vi "SRX Read Velocity Sensor Data.vi"(7 "Target":dbl, 8 "Error":errorcluster, 11 "SRX Ref":T4) -> (0 "Error Out":errorcluster, 2 "Sensor Status Out":T1, 3 "SRX Ref Out":T4)   [LabVIEW 2020, in "Shooter_ACT.lvlib"]
uses:
  Shooter_ACT.lvlib
  <vilib>/Rock Robotics/WPI/MotorControl/WPI_MotorControlDeviceRef.ctl
  <vilib>/Rock Robotics/WPI/MotorControl/WPI_MotorControlType.ctl
  <vilib>/Rock Robotics/SystemInterfaces/DIO/FPGA_DIOPWMChannel.ctl
  <vilib>/Rock Robotics/WPI/PWM/WPI_PWMDeadband.ctl
  <vilib>/Rock Robotics/SystemInterfaces/DIO/FPGA_DIOChannel.ctl
  Cluster_Speed Sensor Values.ctl
  Cluster_Velocity Values.ctl
  Cluster_Voltage Values.ctl
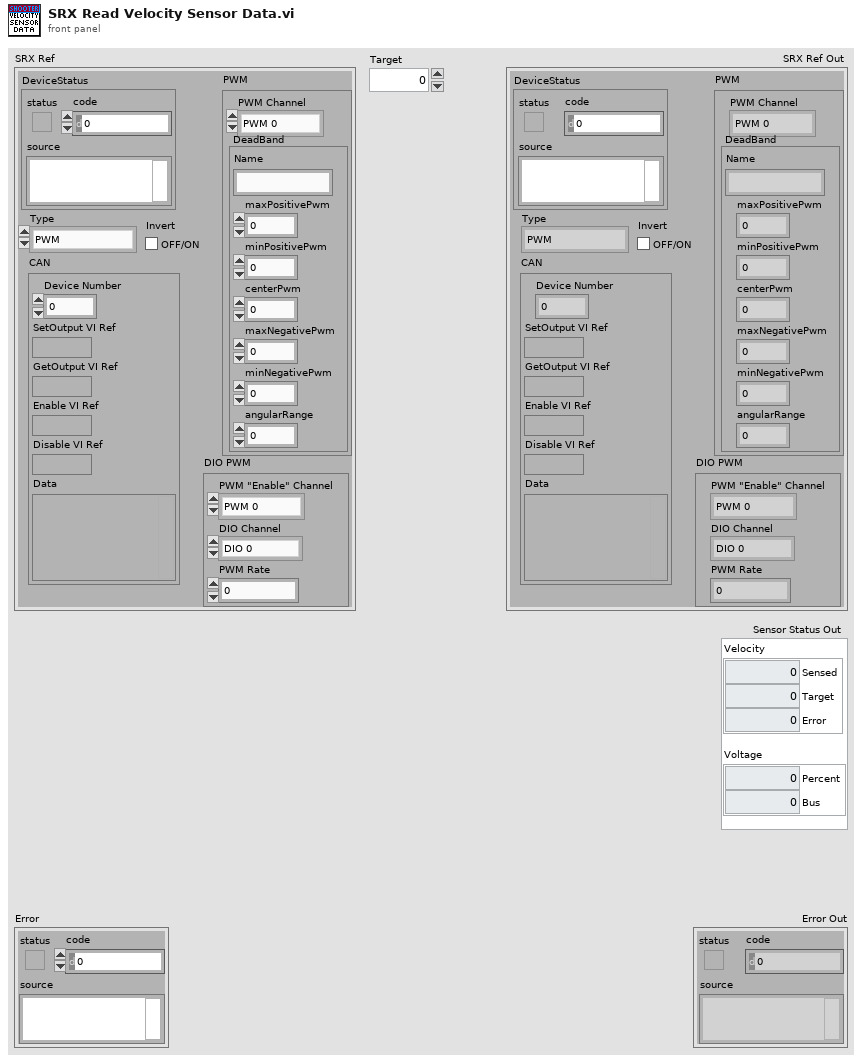
[diagram p1: front panel]
types:
  T1 = typedef "Cluster_Speed Sensor Values.ctl" = cluster{"Velocity":T2, "Voltage":T3}
  T2 = typedef "Shooter_ACT.lvlib/Cluster_Velocity Values.ctl" = cluster{"Sensed":dbl, "Target":dbl, "Error":dbl}
  T3 = typedef "Shooter_ACT.lvlib/Cluster_Voltage Values.ctl" = cluster{"Percent":dbl, "Bus":dbl}
  T4 = typedef "WPI_MotorControlDeviceRef.ctl" = cluster{"DeviceStatus":errorcluster, "Type":T5, "PWM":cluster{"PWM Channel":T6, "DeadBand":T7}, "CAN":cluster{"Device Number":u8, "SetOutput VI Ref":variant, "GetOutput VI Ref":variant, "Enable VI Ref":variant, "Disable VI Ref":variant, "Data":variant}, "Invert":bool, "DIO PWM":cluster{"PWM \"Enable\" Channel":T6, "DIOChannel":T8, "PWM Rate":dbl}}
  T5 = typedef "WPI_MotorControlType.ctl" = enum16{"PWM", "CAN", "DIO PWM"}
  T6 = typedef "FPGA_DIOPWMChannel.ctl" = enum8{"PWM 0", "PWM 1", "PWM 2", "PWM 3", "PWM 4", "PWM 5", "PWM 6", "PWM 7", "PWM 8", "PWM 9", "PWM MXP 0", "PWM MXP 1", "PWM MXP 2", "PWM MXP 3", "PWM MXP 4", "PWM MXP 5", "PWM MXP 6", "PWM MXP 7", "PWM MXP 8", "PWM MXP 9", "Invalid"}
  T7 = typedef "WPI_PWMDeadband.ctl" = cluster{"Name":string, "maxPositivePwm":i32, "minPositivePwm":i32, "centerPwm":i32, "maxNegativePwm":i32, "minNegativePwm":i32, "angularRange":u16}
  T8 = typedef "FPGA_DIOChannel.ctl" = enum8{"DIO 0", "DIO 1", "DIO 2", "DIO 3", "DIO 4", "DIO 5", "DIO 6", "DIO 7", "DIO 8", "DIO 9", "DIO MXP 0", "DIO MXP 1", "DIO MXP 2", "DIO MXP 3", "DIO MXP 4", "DIO MXP 5", "DIO MXP 6", "DIO MXP 7", "DIO MXP 8", "DIO MXP 9", "DIO MXP 10", "DIO MXP 11", "DIO MXP 12", "DIO MXP 13", "DIO MXP 14", "DIO MXP 15", "SPI Port CS1", "SPI Port CS2", "SPI Port CS3", "SPI Port MISO", "SPI Port MOSI", "Invalid"}
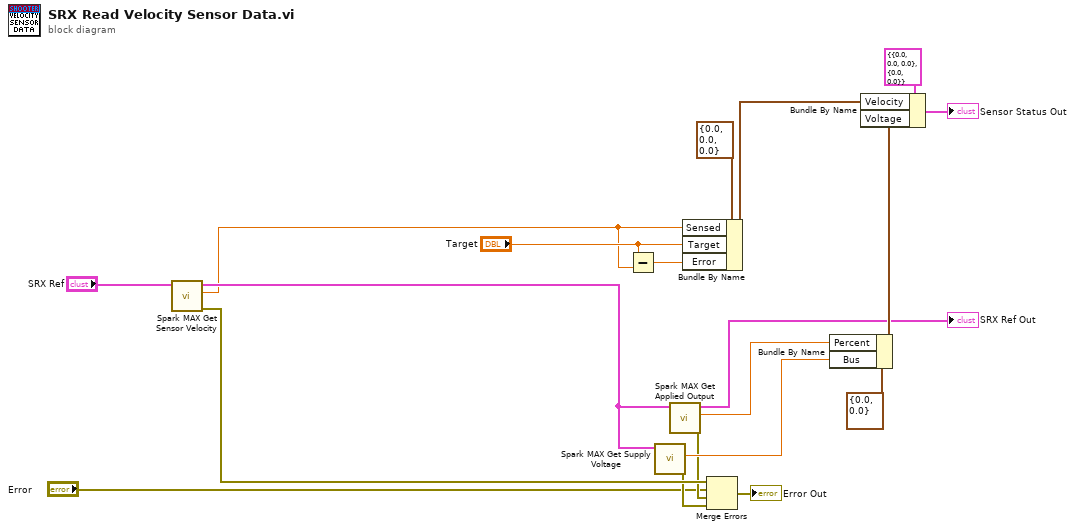
[diagram p0: block diagram]
diagram:
  n1 = call <vilib>:"Spark MAX Get Sensor Velocity.vi"("MotorControlDevRef in"="SRX Ref") -> ("error out"=w11:errorcluster, "Sensor Velocity"=w2:dbl, "MotorControlDevRef out"=w5:T4)  [unwired: 7 in, 1 out]
  n2 = Subtract(x="Target", y=w2) -> (x-y=w1:dbl)
  n3 = call <vilib>:"Spark MAX Get Supply Voltage.vi"("MotorControlDevRef in"=w5) -> ("error out"=w7:errorcluster, "Voltage"=w9:dbl)  [unwired: 7 in, 2 out]
  n4 = call <vilib>:"Spark MAX Get Applied Output.vi"("MotorControlDevRef in"=w5) -> ("error out"=w6:errorcluster, "Applied Output"=w8:dbl, "MotorControlDevRef out"=→"SRX Ref Out":T4)  [unwired: 7 in, 1 out]
  n5 = Bundle By Name(cluster=T2 {"Sensed"=0.0, "Target"=0.0, "Error"=0.0} ("Velocity Data"), "Sensed"=w2, "Target"="Target", "Error"=w1) -> (w14:T2)
  n6 = Merge Errors(w11, "Error", w6, w7) -> (→"Error Out":errorcluster)
  n7 = Bundle By Name(cluster=T3 {"Percent"=0.0, "Bus"=0.0} ("Voltage Data"), "Percent"=w8, "Bus"=w9) -> (w13:T3)
  n8 = Bundle By Name(cluster=T1 {"Velocity"={"Sensed"=0.0, "Target"=0.0, "Error"=0.0}, "Voltage"={"Percent"=0.0, "Bus"=0.0}} ("Sensor Status"), "Velocity"=w14, "Voltage"=w13) -> (→"Sensor Status Out":T1)
